vi "Configure Trigger Model Digital Output Pulse Width.vi"(8 "error in (no error)":errorcluster, 9 "Pulse Width (10 us)":dbl=1e-05, 10 "Digital I/O line   (1)":i32=1 min=1 max=6 step=1 format="%#.6g", 11 "VISA resource name":refnum<visa-resource-name>) -> (0 "error out":errorcluster, 3 "VISA resource name out":refnum<visa-resource-name>)   [LabVIEW 2018, in "Keithley 2450.lvlib"]
doc: "This VI describes the length of time that the trigger line is asserted for output triggers."
uses:
  <instrlib>/Keithley 2450/Keithley 2450.lvlib
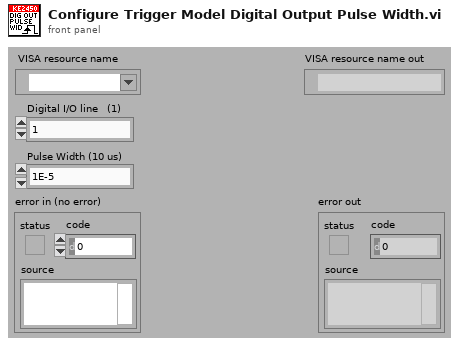
[diagram p1: front panel]
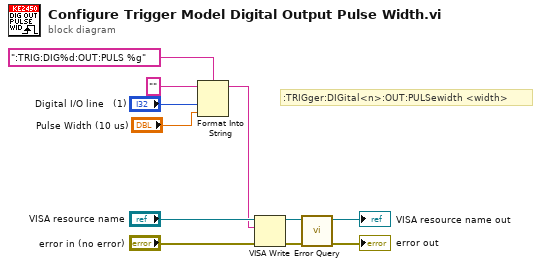
[diagram p0: block diagram]
diagram:
  # ":TRIGger:DIGital<n>:OUT:PULSewidth <width>"
  n1 = Format Into String(format string=":TRIG:DIG%d:OUT:PULS %g", initial string="", "Digital I/O line   (1)", "Pulse Width (10 us)") -> (resulting string=w2:string)  [unwired: 1 in, 1 out]
  n2 = VISA Write(VISA resource name="VISA resource name", write buffer=w2, error in (no error)="error in (no error)") -> (VISA resource name out=w7:refnum<visa-resource-name>, error out=w6:errorcluster)  [unwired: 1 out]
  n3 = call <instrlib>:"Error Query.vi"("error in (no error)"=w6, "VISA resource name"=w7) -> ("error out"=→"error out":errorcluster, "VISA resource name out"=→"VISA resource name out":refnum<visa-resource-name>)  [unwired: 8 out]
